vi "WL Source.vi"(8 "error in (no error)":errorcluster, 11 "VWL (V)":dbl) -> (0 "error out":errorcluster)   [LabVIEW 2019]
uses:
  <vilib>/DAQmx/write.llb/DAQmx Write (Analog 1D DBL NChan 1Samp).vi
  Globals.vi
  <vilib>/DAQmx/create/channels.llb/DAQmx Create Channel (AO-Voltage-Basic).vi
  <vilib>/DAQmx/configure/timing.llb/DAQmx Timing (Sample Clock).vi
  <vilib>/DAQmx/miscellaneous.llb/DAQmx Fill In Error Info.vi
panel:
  out "AO Outputs":dbl[](array[numeric])
  in  "Sample Rate":dbl=1000000.0
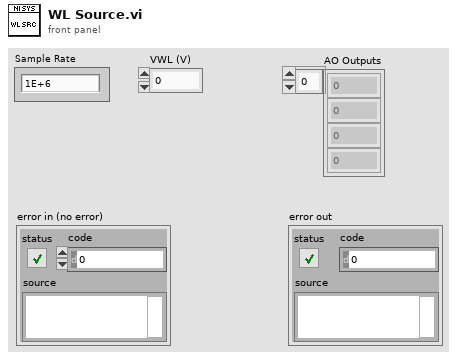
[diagram p1: front panel]
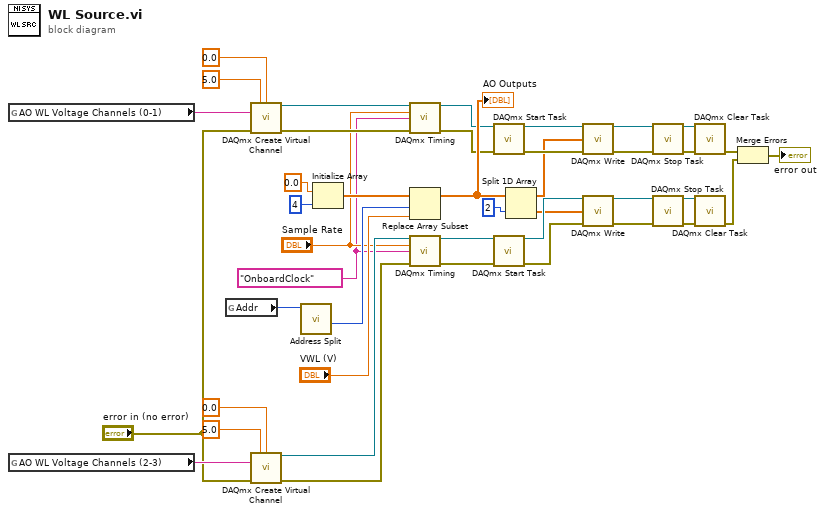
[diagram p0: block diagram]
diagram:
  w6 = tag "OnboardClock" ("Sample Clock Source")
  n1 = global read "Globals.vi" "AO WL Voltage Channels (0-1)"() -> (w17:tag)
  n2 = global read "Globals.vi" "AO WL Voltage Channels (2-3)"() -> (w32:tag)
  n3 = global read "Globals.vi" "Addr"() -> (w38:u16)
  n4 = call-poly <vilib>:"DAQmx Create Virtual Channel.vi"("maximum value"=5.0 ("Max Voltage"), "minimum value"=0.0 ("Min Voltage"), "physical channels"=w17, "error in"="error in (no error)") -> ("task out"=w5:refnum<k21>, "error out"=w16:errorcluster)  [unwired: 10 in]
  n5 = call-poly <vilib>:"DAQmx Create Virtual Channel.vi"("maximum value"=5.0 ("Max Voltage"), "minimum value"=0.0 ("Min Voltage"), "physical channels"=w32, "error in"="error in (no error)") -> ("task out"=w40:refnum<k21>, "error out"=w39:errorcluster)  [unwired: 10 in]
  n6 = call "Address Split.vi"("address"=w38) -> ("wl_ext_sel"=w34:u32)  [unwired: 7 in, 3 out]
  n7 = Initialize Array(0.0 ("element"), 4 ("dimension size")) -> (w35:dbl[])
  n8 = call-poly <vilib>:"DAQmx Timing.vi"("task/channels in"=w5, "rate"="Sample Rate", "source"=w6, "error in"=w16) -> ("task out"=w18:refnum<k21>, "error out"=w19:errorcluster)  [unwired: 10 in]
  n9 = Replace Array Subset(array=w35, new element="VWL (V)", index=w34) -> (w26:dbl[])
  "AO Outputs" <- w26
  n10 = call-poly <vilib>:"DAQmx Timing.vi"("task/channels in"=w40, "rate"="Sample Rate", "source"=w6, "error in"=w39) -> ("task out"=w31:refnum<k21>, "error out"=w30:errorcluster)  [unwired: 10 in]
  n11 = call <vilib>:"DAQmx Start Task.vi"("task/channels in"=w18, "error in"=w19) -> ("task out"=w20:refnum<k21>, "error out"=w21:errorcluster)  [unwired: 12 in]
  n12 = call <vilib>:"DAQmx Start Task.vi"("task/channels in"=w31, "error in"=w30) -> ("task out"=w29:refnum<k21>, "error out"=w28:errorcluster)  [unwired: 12 in]
  n13 = Split 1D Array(array=w26, index=2) -> (first subarray=w7:dbl[], second subarray=w8:dbl[])
  n14 = call-poly <vilib>:"DAQmx Write.vi"("task/channels in"=w20, "data"=w7, "error in"=w21) -> ("task out"=w4:refnum<k21>, "error out"=w3:errorcluster)  [unwired: 10 in, 1 out]
  n15 = call-poly <vilib>:"DAQmx Write.vi"("task/channels in"=w29, "data"=w8, "error in"=w28) -> ("task out"=w2:refnum<k21>, "error out"=w1:errorcluster)  [unwired: 10 in, 1 out]
  n16 = call <vilib>:"DAQmx Stop Task.vi"("task/channels in"=w4, "error in"=w3) -> ("task out"=w23:refnum<k21>, "error out"=w22:errorcluster)  [unwired: 12 in]
  n17 = call <vilib>:"DAQmx Stop Task.vi"("task/channels in"=w2, "error in"=w1) -> ("task out"=w24:refnum<k21>, "error out"=w25:errorcluster)  [unwired: 12 in]
  n18 = call <vilib>:"DAQmx Clear Task.vi"("task in"=w23, "error in"=w22) -> ("error out"=w10:errorcluster)  [unwired: 13 in]
  n19 = call <vilib>:"DAQmx Clear Task.vi"("task in"=w24, "error in"=w25) -> ("error out"=w11:errorcluster)  [unwired: 13 in]
  n20 = Merge Errors(w10, w11) -> (→"error out":errorcluster)
